vi "JS chair get (SubVI).vi"(9 "JS resp":i32, 11 "Telebuf in":u8[](array[numeric])) -> (0 "Auto Depth":bool, 1 "Auto Heading":bool, 2 "t_js_prc":dbl[](array[numeric]), 3 "t_js":dbl[](array[numeric]))   [LabVIEW 2014]
uses:
  <vilib>/imath/engines/lvmath2/RunTimeEngine/Managers/WorkSpace/UID Generator.vi
  <vilib>/imath/engines/lvmath2/RunTimeEngine/RunTimeType/NIMS_RunTimeType_From StrictType (excl LVString).vi
  <instcachedir>/0/NIMS_RunTimeType_From StrictType (excl LVString)_15A5391EEA9C4AACB9955AC755B83D29.lvgen/NIMS_RunTimeType_From StrictType (excl LVString)_15A5391EEA9C4AACB9955AC755B83D29_000.vi
  <vilib>/imath/engines/lvmath2/RunTimeEngine/LocalVariableDefStatement/MC_LocalVariableDefStatement_Display.vi
  <vilib>/imath/engines/lvmath2/RunTimeEngine/RangeToken/NIMS_Range_R2 - Integer.vi
  <instcachedir>/0/NIMS_Range_R2 - Integer_2D1304BAF97744E0A293025746CBADFC.lvgen/NIMS_Range_R2 - Integer_2D1304BAF97744E0A293025746CBADFC_000.vi
  <vilib>/imath/engines/lvmath2/RunTimeEngine/CommandStatement/MC_CommandStatement_break.vi
  <vilib>/imath/engines/lvmath2/RunTimeEngine/IndexRead/NIMS V(S).vi
  <instcachedir>/0/NIMS V(S)_0488751826AF41519A22953C041130DC.lvgen/NIMS V(S)_0488751826AF41519A22953C041130DC_000.vi
  <vilib>/imathl/engines/lvmath/Functions/Error Handling/Create Error.vi
  <vilib>/imath/engines/lvmath2/RunTimeEngine/IndexReplace/NIMS V(S)=S.vi
  <instcachedir>/0/NIMS V(S)=S_2D52C4EC15D8415E870AEE69FB516CCA.lvgen/NIMS V(S)=S_2D52C4EC15D8415E870AEE69FB516CCA_004.vi
  <vilib>/imath/engines/lvmath2/RunTimeEngine/BuiltInFunctions/abs/NIMS_abs(signed).vi
  <instcachedir>/0/NIMS_abs(signed)_C4FCB8E6058B49B797C7C8D53CA5F6EC.lvgen/NIMS_abs(signed)_C4FCB8E6058B49B797C7C8D53CA5F6EC_000.vi
  <instcachedir>/0/NIMS V(S)_0488751826AF41519A22953C041130DC.lvgen/NIMS V(S)_0488751826AF41519A22953C041130DC_002.vi
  <vilib>/imath/engines/lvmath2/RunTimeEngine/ErrorHandling/NIMS_Create Error From Enums.vi
  <instcachedir>/0/NIMS V(S)=S_2D52C4EC15D8415E870AEE69FB516CCA.lvgen/NIMS V(S)=S_2D52C4EC15D8415E870AEE69FB516CCA_000.vi
  <vilib>/imath/engines/lvmath2/RunTimeEngine/BuiltInFunctions/diag/NIMS_diag.vi
  <instcachedir>/0/NIMS_diag_3C4F3DCE8A2D4541A558217542783B22.lvgen/NIMS_diag_3C4F3DCE8A2D4541A558217542783B22_003.vi
  <vilib>/imath/engines/lvmath2/RunTimeEngine/ArithmeticOperatorToken/NIMS_ArithmeticOperator_multmx.vi
  <instcachedir>/0/NIMS_ArithmeticOperator_multmx_CE3986B82B8C4E94A31593A7EF82383B.lvgen/NIMS_ArithmeticOperator_multmx_CE3986B82B8C4E94A31593A7EF82383B_006.vi
  <instcachedir>/0/NIMS_ArithmeticOperator_multmx_CE3986B82B8C4E94A31593A7EF82383B.lvgen/NIMS_ArithmeticOperator_multmx_CE3986B82B8C4E94A31593A7EF82383B_007.vi
  <vilib>/imath/engines/lvmath2/RunTimeEngine/ArithmeticOperatorToken/NIMS_ArithmeticOperator_multmx(M,CV).vi
  <instcachedir>/0/NIMS_ArithmeticOperator_multmx(M,CV)_787B4652E60B4C52835A7FB23671E425.lvgen/NIMS_ArithmeticOperator_multmx(M,CV)_787B4652E60B4C52835A7FB23671E425_000.vi
  <vilib>/imath/engines/lvmath2/RunTimeEngine/VariableToken/NIMS_VariableToken_CondDefinedDefinedByReplace.vi
  <instcachedir>/0/NIMS_VariableToken_CondDefinedDefinedByReplace_D162CFFC24174562A9FEA619A91E1A56.lvgen/NIMS_VariableToken_CondDefinedDefinedByReplace_D162CFFC24174562A9FEA619A91E1A56_002.vi
  <vilib>/imath/engines/lvmath2/RunTimeEngine/IndexRead/NIMS M(S).vi
  <instcachedir>/0/NIMS M(S)_B826C018497E4940AE96BD27B540B6FB.lvgen/NIMS M(S)_B826C018497E4940AE96BD27B540B6FB_000.vi
  <vilib>/imath/engines/lvmath2/RunTimeEngine/NodeEndStatement/NIMS_NodeEndStatement_Get Vector.vi
  <instcachedir>/0/NIMS_NodeEndStatement_Get Vector_00D1625602D843AD9D7EC134A9EC13A2.lvgen/NIMS_NodeEndStatement_Get Vector_00D1625602D843AD9D7EC134A9EC13A2_001.vi
  <vilib>/imath/engines/lvmath2/RunTimeEngine/VariableToken/NIMS_VariableToken_CondDefined.vi
  <instcachedir>/0/NIMS_VariableToken_CondDefined_EE8DD211A89249938CE6537267F5C9B3.lvgen/NIMS_VariableToken_CondDefined_EE8DD211A89249938CE6537267F5C9B3_003.vi
  <vilib>/imath/engines/lvmath/Functions/Error Handling/MergeErrorsWrapper.vi
  <vilib>/imath/engines/lvmath2/RunTimeEngine/Managers/SymbolTable/Clear UID.vi
  <vilib>/imath/engines/lvmath2/RunTimeEngine/NodeEndStatement/NIMS_NodeEndStatement_Output.vi
  <instcachedir>/0/NIMS_NodeEndStatement_Output_53EC0D466D134D7ABD903AC30B43404B.lvgen/NIMS_NodeEndStatement_Output_53EC0D466D134D7ABD903AC30B43404B_005.vi
  <vilib>/imath/engines/lvmath2/RunTimeEngine/ErrorHandling/NIMS_Finalize Error.vi
  <vilib>/imath/engines/lvmath2/RunTimeEngine/Managers/SymbolTable/NIMS_WorkSpace.lvlib
panel:
  out "Z_2":u32
  out "Y_2  (side)":u32
  out "X_2  (vert)":u32
  out "Z_1":u32
  out "X_1 (turn)":u32
  out "Y_1 (forward)":u32
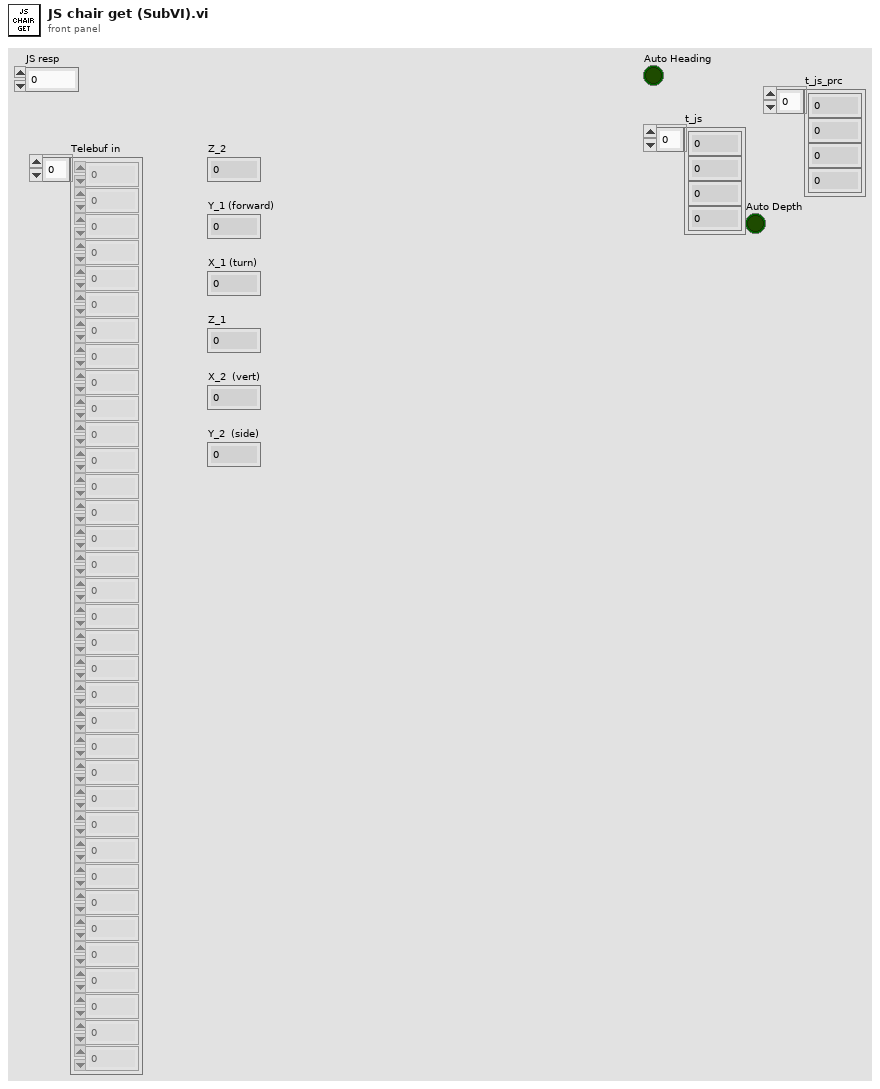
[diagram p1: front panel]
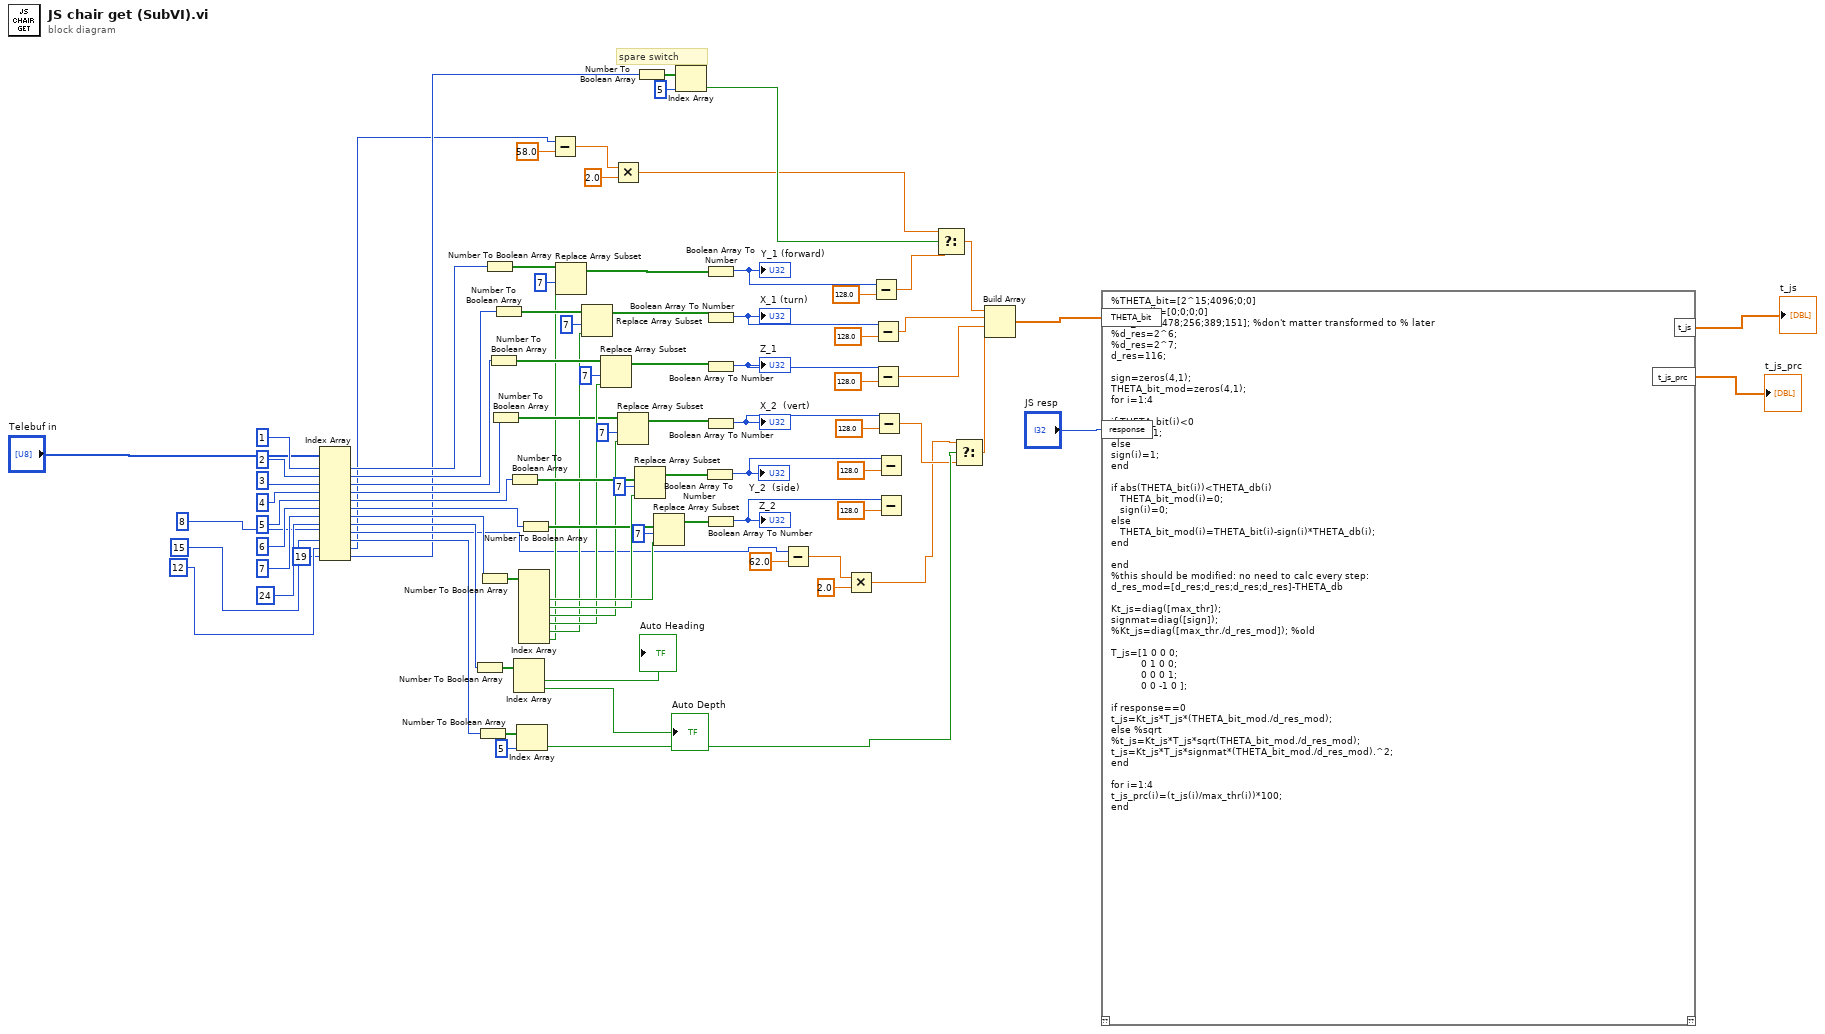
[diagram p0: block diagram]
diagram:
  # "spare switch"
  n1 = Index Array(array="Telebuf in", index #1=1 ("index"), index #2=2 ("index"), index #3=3 ("index"), index #4=4 ("index"), index #5=5 ("index"), index #6=6 ("index"), index #7=7 ("index"), index #8=24 ("index"), index #9=8 ("index"), index #10=15 ("index"), index #11=12 ("index"), index #12=19 ("index")) -> (element #1=w58:u8, element #2=w82:u8, element #3=w72:u8, element #4=w77:u8, element #5=w83:u8, element #6=w89:u8, element #7=w60:u8, element #8=w30:u8, element #9=w20:u8, element #10=w24:u8, element #11=w5:u8, element #12=w9:u8)
  n2 = Number To Boolean Array(number=w30) -> (Boolean array=w31:bool[])
  n3 = Number To Boolean Array(number=w24) -> (Boolean array=w25:bool[])
  n4 = Number To Boolean Array(number=w60) -> (Boolean array=w61:bool[])
  n5 = Number To Boolean Array(number=w58) -> (Boolean array=w59:bool[])
  n6 = Number To Boolean Array(number=w72) -> (Boolean array=w69:bool[])
  n7 = Number To Boolean Array(number=w77) -> (Boolean array=w75:bool[])
  n8 = Number To Boolean Array(number=w82) -> (Boolean array=w67:bool[])
  n9 = Number To Boolean Array(number=w83) -> (Boolean array=w79:bool[])
  n10 = Index Array(array=w31) -> (element #1=→"Auto Heading":bool, element #2=→"Auto Depth":bool)  [unwired: 2 in]
  n11 = Index Array(array=w25, index=5) -> (element=w22:bool)
  n12 = Index Array(array=w61) -> (element #2=w88:bool, element #3=w87:bool, element #4=w78:bool, element #5=w76:bool, element #6=w68:bool, element #7=w62:bool)  [unwired: 7 in, 1 out]
  n13 = Number To Boolean Array(number=w89) -> (Boolean array=w86:bool[])
  n14 = Subtract(x=w5, y=58.0) -> (x-y=w8:dbl)
  n15 = Replace Array Subset(array=w59, new element=w62, index=7) -> (w64:bool[])
  n16 = Replace Array Subset(array=w67, new element=w68, index=7) -> (w65:bool[])
  n17 = Replace Array Subset(array=w69, new element=w76, index=7) -> (w71:bool[])
  n18 = Multiply(x=w8, y=2.0) -> (x*y=w3:dbl)
  n19 = Replace Array Subset(array=w75, new element=w78, index=7) -> (w73:bool[])
  n20 = Replace Array Subset(array=w79, new element=w87, index=7) -> (w81:bool[])
  n21 = Number To Boolean Array(number=w9) -> (Boolean array=w10:bool[])
  n22 = Replace Array Subset(array=w86, new element=w88, index=7) -> (w84:bool[])
  n23 = Index Array(array=w10, index=5) -> (element=w4:bool)
  n24 = Boolean Array To Number(Boolean array=w81) -> (number=w39:u32)
  "Y_2  (side)" <- w39
  n25 = Boolean Array To Number(Boolean array=w64) -> (number=w49:u32)
  "Y_1 (forward)" <- w49
  n26 = Boolean Array To Number(Boolean array=w65) -> (number=w42:u32)
  "X_1 (turn)" <- w42
  n27 = Boolean Array To Number(Boolean array=w71) -> (number=w41:u32)
  "Z_1" <- w41
  n28 = Boolean Array To Number(Boolean array=w73) -> (number=w40:u32)
  "X_2  (vert)" <- w40
  n29 = Boolean Array To Number(Boolean array=w84) -> (number=w38:u32)
  "Z_2" <- w38
  n30 = Subtract(x=w20, y=62.0) -> (x-y=w15:dbl)
  n31 = Multiply(x=w15, y=2.0) -> (x*y=w14:dbl)
  n32 = Subtract(x=w49, y=128.0) -> (x-y=w2:dbl)
  n33 = Subtract(x=w42, y=128.0) -> (x-y=w37:dbl)
  n34 = Subtract(x=w41, y=128.0) -> (x-y=w36:dbl)
  n35 = Subtract(x=w40, y=128.0) -> (x-y=w19:dbl)
  n36 = Subtract(x=w39, y=128.0) -> ()  [unwired: 1 out]
  n37 = Subtract(x=w38, y=128.0) -> ()  [unwired: 1 out]
  n38 = Select(t=w3, s=w4, f=w2) -> (s? t:f=w1:dbl)
  n39 = Select(t=w14, s=w22, f=w19) -> (s? t:f=w18:dbl)
  n40 = Build Array(w1, w37, w36, w18) -> (w35:dbl[])
  n41 = mathscript code="%THETA_bit=[2^15;4096;0;0]\nTHETA_db=[0;0;0;0]\nmax_thr=[478;256;389;151]; %don't matter transformed to % later\n%d_res=2^6;\n%d_res=2^7;\nd_res=116;\n\nsign=zeros(4,1);\nTHETA_bit_mod=zeros(4,1);\nfor i=1:4\n \nif THETA_bit(i)<0\nsign(i)=-1;   \nelse\nsign(i)=1;    \nend\n    \nif abs(THETA_bit(i))<THETA_db(i)\n   THETA_bit_mod(i)=0;\n   sign(i)=0;\nelse\n   THETA_bit_mod(i)=THETA_bit(i)-sign(i)*THETA_db(i);\nend\n\nend\n%this should be modified: no need to calc every step:\nd_res_mod=[d_res;d_res;d_res;d_res]-THETA_db\n\nKt_js=diag([max_thr]);\nsignmat=diag([sign]);\n%Kt_js=diag([max_thr./d_res_mod]); %old\n\nT_js=[1 0 0 0;\n          0 1 0 0;\n          0 0 0 1;\n          0 0 -1 0 ];\n\nif response==0\nt_js=Kt_js*T_js*(THETA_bit_mod./d_res_mod);\nelse %sqrt\n%t_js=Kt_js*T_js*sqrt(THETA_bit_mod./d_res_mod);\nt_js=Kt_js*T_js*signmat*(THETA_bit_mod./d_res_mod).^2;\nend\n\nfor i=1:4\nt_js_prc(i)=(t_js(i)/max_thr(i))*100;\nend"("THETA_bit"=w35, "response"="JS resp") -> ("t_js"=→"t_js":dbl[], "t_js_prc"=→"t_js_prc":dbl[])  [unwired: 1 in, 1 out]
